vi "emi_Get Debug Log status.vi"(9 "error in (no error)":errorcluster) -> (8 "Debug Log":bool, 10 "error out":errorcluster)   [LabVIEW 2011]
doc: "Checks wheter the application id closeing,"
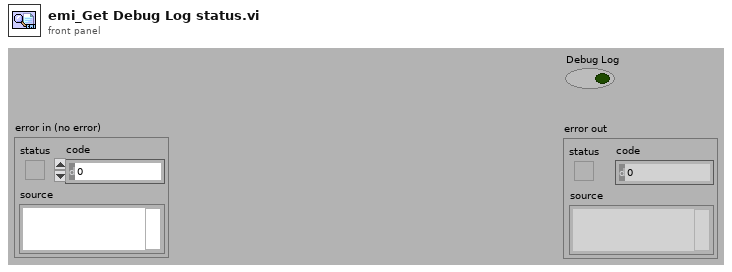
[diagram p1: front panel]
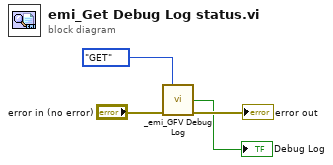
[diagram p0: block diagram]
diagram:
  n1 = call "_emi_GFV Debug Log.vi"("Action(GET)"=enum16{"GET", "SET"}."GET", "error in (no error)"="error in (no error)") -> ("Debug Log out"=→"Debug Log":bool, "error out"=→"error out":errorcluster)  [unwired: 12 in]
